vi "Set Entry Position.vi"(8 "error in (no error)":errorcluster, 10 "Station":T1, 11 "Car Wash Controller in":refnum<class "Car Wash Controller.lvclass">) -> (0 "error out":errorcluster, 3 "Car Wash Controller out":refnum<class "Car Wash Controller.lvclass">)   [LabVIEW 2019, in "Car Wash Controller.lvlib" / "Car Wash Controller.lvclass"]
uses:
  Car Wash Controller.lvclass
  Vehicle Position Simulation Actor/Car Wash Controller/Station -Enum.ctl
  Car Wash Controller.lvclass/Car Wash Controller.ctl
  Vehicle Position Simulation Actor/Vehicle Position Simulation Actor Messages/Write Vehicle Position Msg/Write Vehicle Position Msg.lvclass/Write Vehicle Position Msg.ctl
  <vilib>/ActorFramework/Message Enqueuer/Message Enqueuer.lvclass/Message Enqueuer.ctl
  <vilib>/ActorFramework/Message Enqueuer/Enqueue.vi
  Vehicle Position Simulation Actor/Vehicle Position Simulation Actor Messages/Write Vehicle Position Msg/Write Vehicle Position Msg.lvclass
  C:/Program Files (x86)/National Instruments/LabVIEW 2019/vi.lib/ActorFramework/Message/Message.lvclass
  <vilib>/ActorFramework/Message Priority Queue/Priority Enqueue.vi
  Vehicle Position Simulation Actor/Car Wash Controller/Vehicle Position Simulation Actor.lvclass
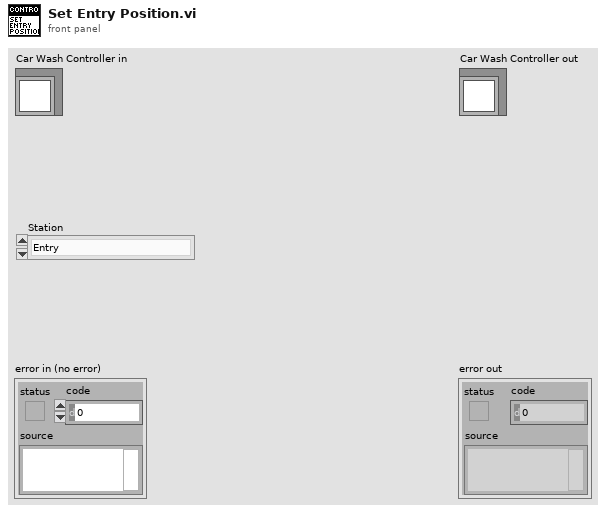
[diagram p1: front panel]
types:
  T1 = typedef "Vehicle Position Sinmulation Actor.lvlib/Vehicle Position Simulation Actor.lvclass/Station -Enum.ctl" = enum16{"Entry", "Station1", "Station2", "Station3", "Exit"}
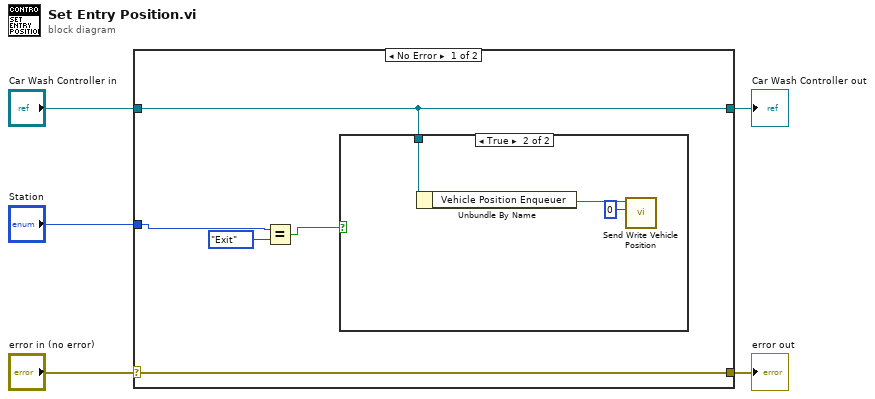
[diagram p0: block diagram]
diagram:
  n1 = case shown="No Error" "error in (no error)" {
    selector: "error in (no error)" -> [w10 w15]
    tunnel: [w10 w15] -> w4
    tunnel: [w9 w14] -> w2
    tunnel: "Car Wash Controller in" -> [w9 w14]
    tunnel: "Station" -> [w8 _]
    frame No Error {
      n2 = Equal?(x=w8, y=Station_-Enum."Exit") -> (x = y?=w6:bool)
      n3 = case shown="True" w6 {
        tunnel: w9 -> [_ w13]
        frame False {
        }
        frame True {
          n4 = Unbundle By Name(w13) -> ("Vehicle Position Enqueuer"=w12:refnum<class "Message Enqueuer.lvclass">)
          n5 = call "Send Write Vehicle Position.vi"("Vehicle Position Simulation"=u8 0, "Message Enqueuer"=w12) -> ()  [unwired: 8 in, 2 out]
        }
      }
    }
    frame Error {
    }
  }
  "error out" <- w4
  "Car Wash Controller out" <- w2
